vi "Exemple2.vi"() -> ()   [LabVIEW 2019]
uses:
  support/TPC-Enum.ctl
  support/Global 1.vi
panel:
  out "Numeric":i32
  in  "Tab Control":enum32{"Page 1", "Page 2"}(tab)
  in  "Boolean Button":bool
  in  "Enum Test":u16(ring) items=["Enum 0", "Enum 1", "Enum 2"]
  in  "Play Button":bool
  in  "Test request":string
  out "TCP loop status":T1
  out "Main Loop Status":string
  out "Labview response":string
  out "Received request":string
  in  "Exit Button":bool
  in  "Numeric Control U16":u16
  in  "Numeric Control DBL":dbl
  # "Main Vi Example"
  # "Debug section"
  # "TCP-Communication Vi Input"
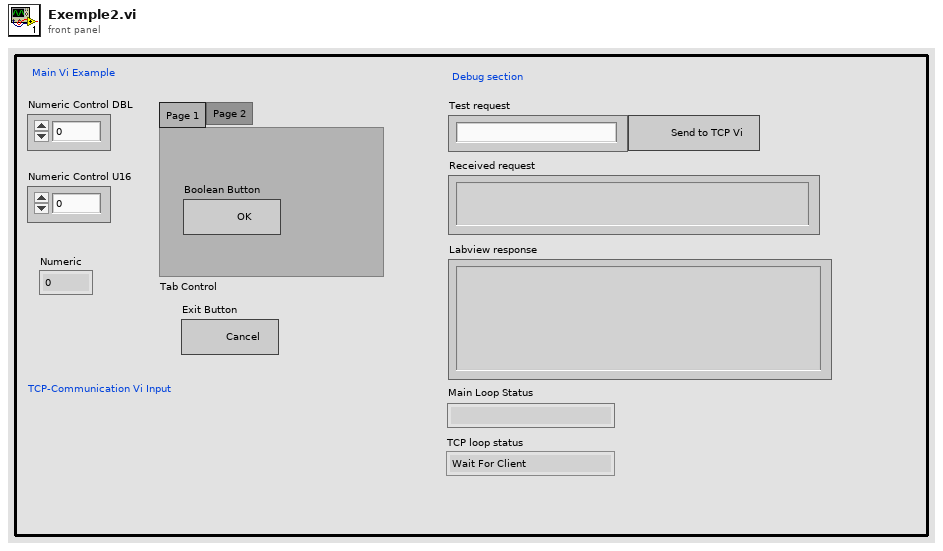
[diagram p1: front panel]
types:
  T1 = typedef "TPC-Enum.ctl" = enum16{"Wait For Client", "Check Client", "Listen"}
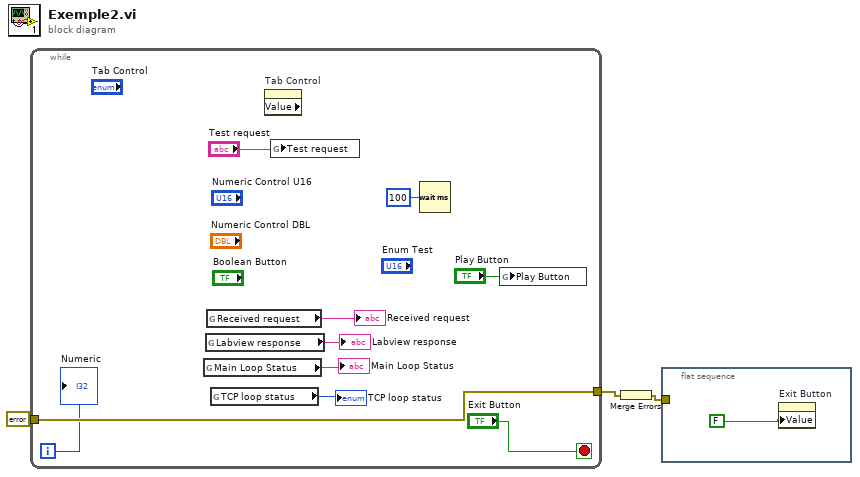
[diagram p0: block diagram]
diagram:
  n1 = while {
    tunnel: errorcluster {"status"=FALSE, "code"=0, "source"=""} ("error out") -> [w5]
    tunnel: [w5] -> w2
    i -> [w4]
    stop <- "Exit Button" stop-if-true
    n2 = global read "Global 1.vi" "Main Loop Status"() -> (→"Main Loop Status":string)
    n3 = global read "Global 1.vi" "Labview response"() -> (→"Labview response":string)
    n4 = global read "Global 1.vi" "Received request"() -> (→"Received request":string)
    n5 = global read "Global 1.vi" "TCP loop status"() -> (→"TCP loop status":T1)
    n6 = property on="Tab Control" class="TabCtl (strict)" props=["Value"]() -> ()  [unwired: 2 in, 3 out]
    n7 = global write "Global 1.vi" "Test request"("Test request") -> ()
    n8 = Wait (ms)(milliseconds to wait=u32 100) -> ()  [unwired: 1 out]
    n9 = global write "Global 1.vi" "Play Button"("Play Button") -> ()
    "Numeric" <- w4
  }
  n10 = Merge Errors(w2) -> (w1:errorcluster)
  n11 = flat-sequence {
    tunnel: w1 -> [_]
    frame #0 {
      n12 = property on="Exit Button" class="Bool (strict)"("Value"=FALSE ("Exit Button")) -> ()  [unwired: 2 in, 2 out]
    }
  }
